vi "CalcRotationAngles.vi"(0 "StrafeAngle":dbl, 5 "StrafeMagnitude":dbl, 7 "ZAxis":dbl, 9 "XAxis":dbl, 11 "YAxis":dbl) -> (4 "Angles":dbl[](array[numeric]), 6 "Speeds":dbl[](array[numeric]))   [LabVIEW 2018]
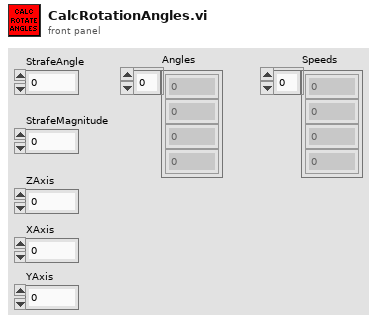
[diagram p1: front panel]
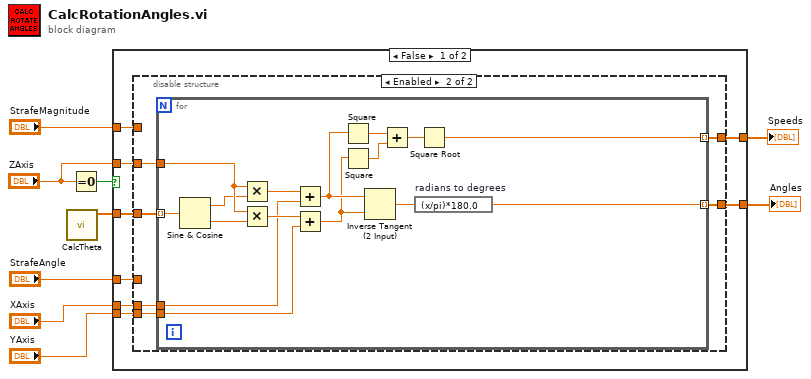
[diagram p0: block diagram]
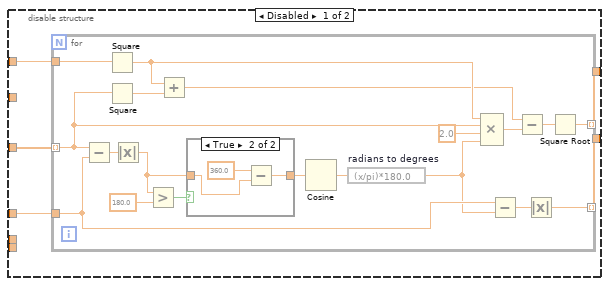
[diagram p2: hidden frame]
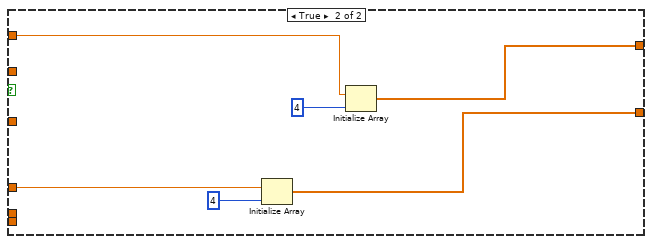
[diagram p4: hidden frame]
diagram:
  n1 = call "CalcTheta.vi"() -> ("ThetaValues"=w3:dbl[])  [unwired: 11 in]
  n2 = Equal To 0?(x="ZAxis") -> (x = 0?=w6:bool)
  n3 = case shown="False" w6 {
    tunnel: "StrafeAngle" -> [w17 w69]
    tunnel: [w16 w68] -> w2
    tunnel: "StrafeMagnitude" -> [w15 w71]
    tunnel: [w14 w70] -> w7
    tunnel: w3 -> [w13 _]
    tunnel: "XAxis" -> [w12 _]
    tunnel: "YAxis" -> [w11 _]
    tunnel: "ZAxis" -> [w10 _]
    frame False {
      n4 = disable-structure shown="Enabled" {
        disable-tunnel: w17 -> [w22 _]
        disable-tunnel: [w21 w47] -> w16
        disable-tunnel: w15 -> [w20 _]
        disable-tunnel: [w19 w46] -> w14
        disable-tunnel: w13 -> [w18 w51]
        disable-tunnel: w12 -> [_ w49]
        disable-tunnel: w11 -> [_ w48]
        disable-tunnel: w10 -> [_ w50]
        frame Disabled {
          n5 = for {
            tunnel: w18 -> [w25] mode=indexing
            tunnel: w22 -> [w27]
            tunnel: w20 -> [w35]
            tunnel: [w23] -> w19 mode=indexing
            tunnel: [w29] -> w21 mode=indexing
            n6 = Subtract(x=w25, y=w27) -> (x-y=w30:dbl)
            n7 = Square(x=w35) -> (x^2=w33:dbl)
            n8 = Square(x=w25) -> (x^2=w34:dbl)
            n9 = Absolute Value(x=w30) -> (abs(x)=w39:dbl)
            n10 = Greater?(x=w39, y=180.0) -> (0:w41:bool)
            n11 = Add(x=w33, y=w34) -> (x+y=w32:dbl)
            n12 = case shown="True" w41 {
              tunnel: w39 -> [w42 w43]
              tunnel: [w42 w44] -> w37
              frame False {
              }
              frame True {
                n13 = Subtract(x=360.0, y=w43) -> (x-y=w44:dbl)
              }
            }
            n14 = Cosine(x=w37) -> (cos(x)=w36:dbl)
            n15 = expression code="(x/pi)*180.0" "radians to degrees"(w36) -> (w26:dbl)
            n16 = Compound Arithmetic op=MULTIPLY(w33, w25, 2.0 ("value"), w26) -> (w31:dbl)
            n17 = Subtract(x=w27, y=w26) -> (x-y=w28:dbl)
            n18 = Subtract(x=w32, y=w31) -> (x-y=w24:dbl)
            n19 = Absolute Value(x=w28) -> (abs(x)=w29:dbl)
            n20 = Square Root(x=w24) -> (sqrt(x)=w23:dbl)
          }
        }
        frame Enabled {
          n21 = for {
            tunnel: w51 -> [w67] mode=indexing
            tunnel: w50 -> [w66]
            tunnel: w49 -> [w53]
            tunnel: w48 -> [w52]
            tunnel: [w56] -> w47 mode=indexing
            tunnel: [w57] -> w46 mode=indexing
            n22 = Sine & Cosine(0:w67) -> (1:w54:dbl, 2:w55:dbl)
            n23 = Multiply(x=w66, y=w54) -> (x*y=w64:dbl)
            n24 = Multiply(x=w66, y=w55) -> (x*y=w65:dbl)
            n25 = Add(x=w64, y=w53) -> (x+y=w62:dbl)
            n26 = Add(x=w65, y=w52) -> (x+y=w61:dbl)
            n27 = Square(x=w62) -> (x^2=w60:dbl)
            n28 = Square(x=w61) -> (x^2=w59:dbl)
            n29 = Inverse Tangent (2 Input)(1:w61, 2:w62) -> (0:w63:dbl)
            n30 = Add(x=w60, y=w59) -> (x+y=w58:dbl)
            n31 = expression code="(x/pi)*180.0" "radians to degrees"(w63) -> (w56:dbl)
            n32 = Square Root(x=w58) -> (sqrt(x)=w57:dbl)
          }
        }
      }
    }
    frame True {
      n33 = Initialize Array(w69, 4 ("dimension size")) -> (w68:dbl[])
      n34 = Initialize Array(w71, 4 ("dimension size")) -> (w70:dbl[])
    }
  }
  "Angles" <- w2
  "Speeds" <- w7
